vi "AH_OpenFile.vi"(7 "Status Ref":refnum<vi>, 8 "error in":errorcluster, 10 "Config_Cluster":T1={"General"={"Config.ini"=path "", "Default Logging Path"=path ""}, "Hardware"={"Global T VAR"="", "Global B VAR"="", "VISAS"={"GEN COM"="", "SCOPE COM"="", "VNA COM"=""}, "Connected?"={"SCOPE"=FALSE, "GEN"=FALSE, "VNA"=FALSE}}, "Operation"={"Operation Mode"=enum."Idle-Off", "Status"="", "NewLog?"=FALSE, "OvenWarn"=FALSE, "Scope Settings"={"TimeBase"=0.0, "VerticalScale"=4.0}}}) -> (0 "error out":errorcluster, 2 "Config_Cluster Out":T1={"General"={"Config.ini"=path "", "Default Logging Path"=path ""}, "Hardware"={"Global T VAR"="", "Global B VAR"="", "VISAS"={"GEN COM"="", "SCOPE COM"="", "VNA COM"=""}, "Connected?"={"SCOPE"=FALSE, "GEN"=FALSE, "VNA"=FALSE}}, "Operation"={"Operation Mode"=enum."Idle-Off", "Status"="", "NewLog?"=FALSE, "OvenWarn"=FALSE, "Scope Settings"={"TimeBase"=0.0, "VerticalScale"=4.0}}}, 3 "refnum out":refnum<file>, 4 "FileOpen?":bool)   [LabVIEW 2021]
uses:
  Config_Cluster.ctl
  Mode_Enum.ctl
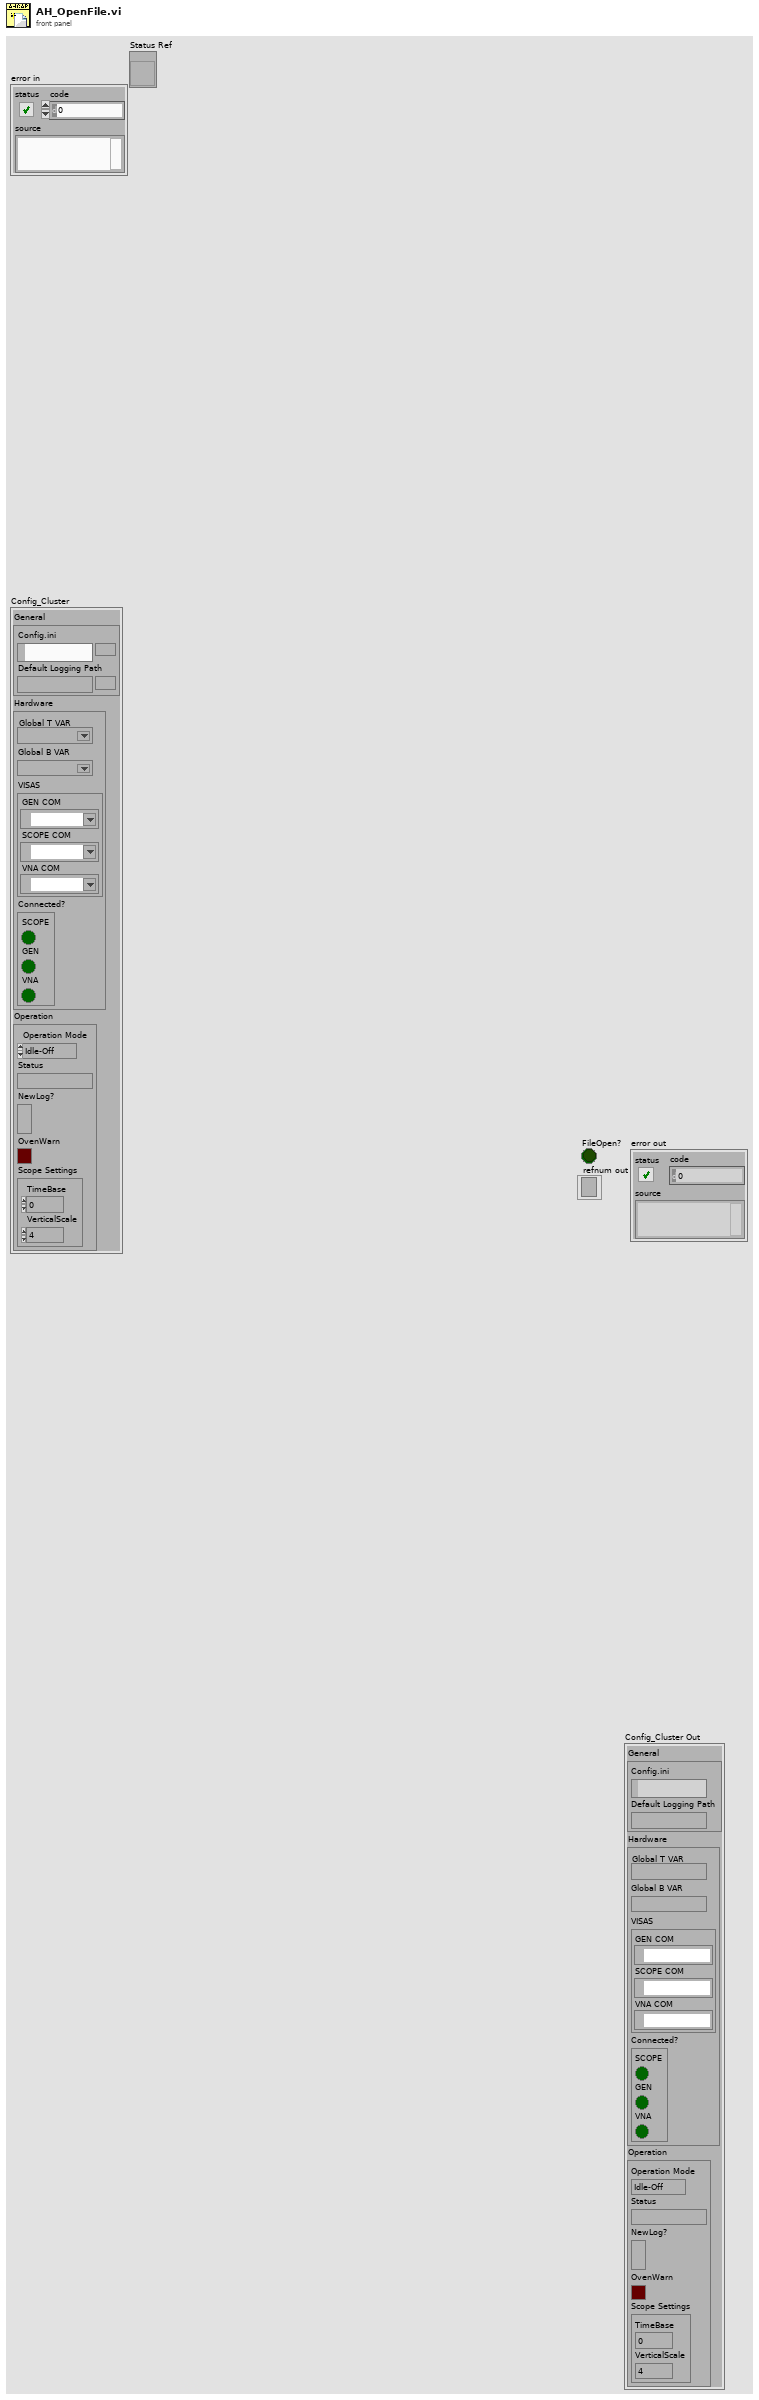
[diagram p1: front panel]
types:
  T1 = typedef "Config_Cluster.ctl" = cluster{"General":cluster{"Config.ini":path, "Default Logging Path":path}, "Hardware":cluster{"Global T VAR":refnum<k21>, "Global B VAR":refnum<k21>, "VISAS":cluster{"GEN COM":refnum<visa-resource-name>, "SCOPE COM":refnum<visa-resource-name>, "VNA COM":refnum<visa-resource-name>}, "Connected?":cluster{"SCOPE":bool, "GEN":bool, "VNA":bool}}, "Operation":cluster{"Operation Mode":T2, "Status":string, "NewLog?":bool, "OvenWarn":bool, "Scope Settings":cluster{"TimeBase":dbl, "VerticalScale":dbl}}}
  T2 = typedef "Mode_Enum.ctl" = enum16{"Logging", "Idle-Off", "Idle"}
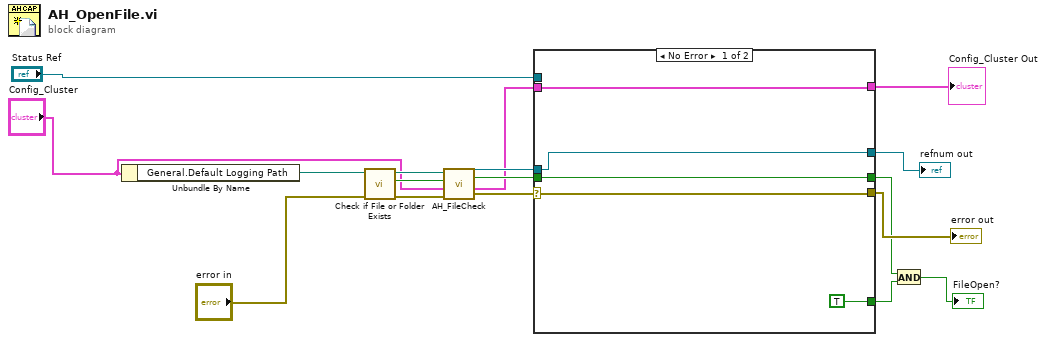
[diagram p0: block diagram]
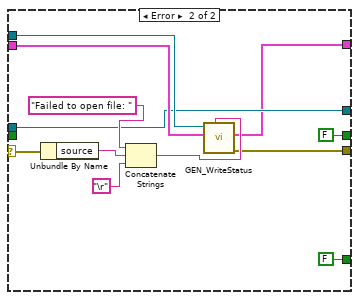
[diagram p2: hidden frame]
diagram:
  n1 = Unbundle By Name("Config_Cluster") -> ("General.Default Logging Path"=w15:path)
  n2 = call <vilib>:"Check if File or Folder Exists.vi"("error in (no error)"="error in", "path"=w15) -> ("error out"=w9:errorcluster, "file or folder exists?"=w10:bool, "dup path"=w11:path)  [unwired: 7 in]
  n3 = call "AH_FileCheck.vi"("error in"=w9, "Config_Cluster"="Config_Cluster", "Exists"=w10, "Path IN"=w11) -> ("error Out"=w6:errorcluster, "Config_Cluster Out"=w1:T1, "Continue"=w7:bool, "refnum"=w8:refnum<file>)  [unwired: 4 in]
  n4 = case shown="No Error" w6 {
    selector: w6 -> [w22 w32]
    tunnel: w8 -> [w21 w26]
    tunnel: "Status Ref" -> [_ w34]
    tunnel: w1 -> [w19 w33]
    tunnel: [w22 w27] -> w13
    tunnel: [w21 w26] -> w14
    tunnel: [TRUE FALSE] -> w4
    tunnel: [w19 w24] -> w12
    tunnel: w7 -> [w18 _]
    tunnel: [w18 FALSE ("Continue")] -> w3
    frame No Error {
    }
    frame Error {
      n5 = Unbundle By Name(w32) -> ("source"=w30:string)
      n6 = Concatenate Strings("Failed to open file: " ("string"), w30, "\r") -> (w28:string)
      n7 = call "GEN_WriteStatus.vi"("Input String"=w28, "Config_Cluster"=w33, "Status Ref"=w34) -> ("error out"=w27:errorcluster, "Config_Cluster Out"=w24:T1)  [unwired: 7 in]
    }
  }
  "refnum out" <- w14
  "error out" <- w13
  "Config_Cluster Out" <- w12
  n8 = And(x=w3, y=w4) -> (x .and. y?=→"FileOpen?":bool)
